vi "SetStartBitFromLabview.vi"(11 "input bool array":bool[](array[boolean])) -> (3 "output bool array":bool[](array[boolean]))   [LabVIEW 2020]
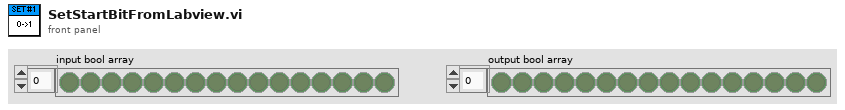
[diagram p1: front panel]
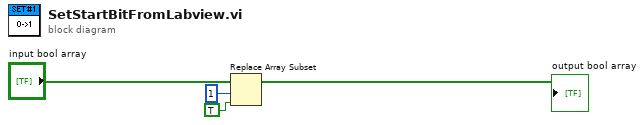
[diagram p0: block diagram]
diagram:
  n1 = Replace Array Subset(array="input bool array", new element=TRUE ("new element/subarray"), index=1) -> (→"output bool array":bool[])
